vi "test.vi"(8 "error in (no error)":errorcluster, 11 "RSA in":refnum<class "RSA.lvclass">) -> (0 "error out":errorcluster, 3 "RSA out":refnum<class "RSA.lvclass">)   [LabVIEW 2012, in "RSA.lvclass"]
uses:
  RSA.lvclass
panel:
  out "actuator out":dbl
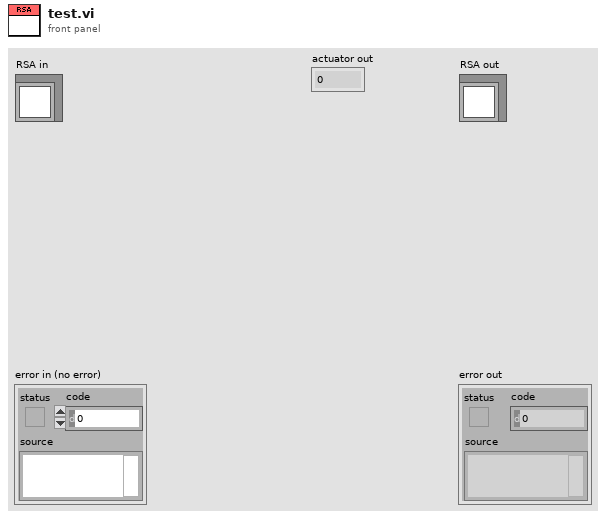
[diagram p1: front panel]
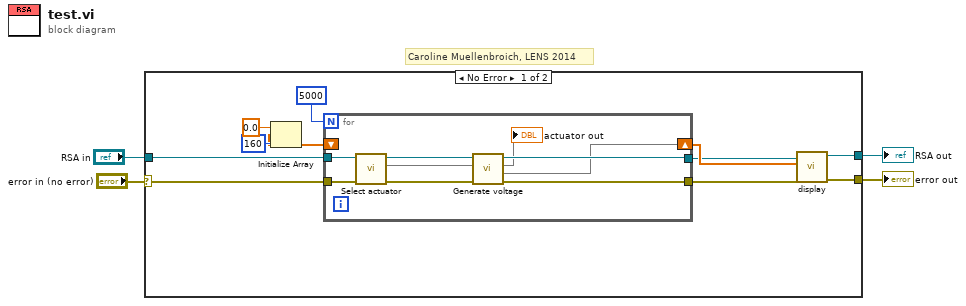
[diagram p0: block diagram]
diagram:
  # "Caroline Muellenbroich, LENS 2014"
  n1 = case shown="No Error" "error in (no error)" {
    selector: "error in (no error)" -> [w15 w25]
    tunnel: [w10 w26] -> w2
    tunnel: "RSA in" -> [w13 w26]
    tunnel: [w11 w25] -> w1
    frame No Error {
      n2 = Initialize Array(0.0 ("element"), 160 ("dimension size")) -> (w7:dbl[])
      n3 = for {
        N: 5000 -> [_]
        tunnel: w13 -> [w24]
        tunnel: w15 -> [w23]
        shift-right: [w18] -> w12
        shift-left: w7 -> [_]
        tunnel: [w20] -> w6
        tunnel: [w19] -> w5
        n4 = call-dynamic "Select actuator.vi"("error in (no error)"=w23, "RSA in"=w24) -> ("error out"=w21:errorcluster, 2:w17, "RSA out"=w22:refnum<class "RSA.lvclass">)  [unwired: 7 in]
        n5 = call "Generate voltage.vi"("error in (no error)"=w21, 10:w17, "RSA in"=w22) -> ("error out"=w19:errorcluster, 1:w18, 2:→"actuator out", "RSA out"=w20:refnum<class "RSA.lvclass">)  [unwired: 5 in]
      }
      n6 = call-dynamic "display.vi"("error in (no error)"=w5, "current plus 1 in"=w12, "RSA in"=w6) -> ("error out"=w11:errorcluster, "RSA out"=w10:refnum<class "RSA.lvclass">)  [unwired: 7 in]
    }
    frame Error {
    }
  }
  "error out" <- w1
  "RSA out" <- w2
